vi "StoreClassesPaths.vi"(8 "error in":errorcluster, 10 "start path":path, 11 "Repository in":refnum<class "NISE_CEF_Repository.lvclass">) -> (0 "error out":errorcluster, 3 "Repository out":refnum<class "NISE_CEF_Repository.lvclass">)   [LabVIEW 2013, in "NISE_CEF_Repository.lvclass"]
doc: "Stores the paths and classes name that the repo use.\n The default behavior is to store the path to the main folder containing the classes. If a more complex file structure is required this file needs to find all the classes and store the name and path pairs."
uses:
  NISE_CEF_Repository.lvclass
  class discovery singleton/class discovery singleton methods.ctl
  class discovery singleton/class discovery singleton.lvlib
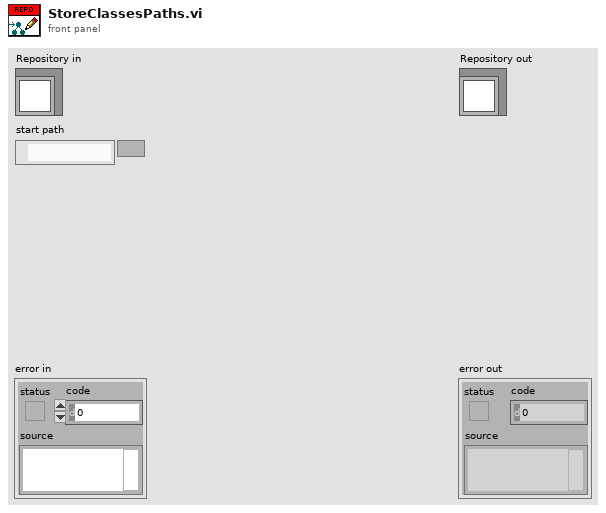
[diagram p1: front panel]
types:
  T1 = typedef "class discovery singleton.lvlib/class discovery singleton methods.ctl" = enum16{"add search paths", "load class by name", "list available classes", "get class path"}
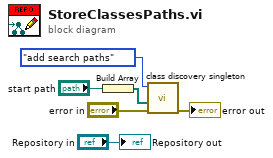
[diagram p0: block diagram]
diagram:
  n1 = Build Array("start path") -> (w3:path[])
  n2 = call "class discovery singleton.vi"("error in"="error in", "Plugin Search Paths"=w3, "method"=class_discovery_singleton_methods."add search paths") -> ("error out"=→"error out":errorcluster)  [unwired: 5 in, 3 out]
  "Repository out" <- "Repository in"
